vi "Run with Subpanel Settings.vi"(8 "error in (no error)":errorcluster, 11 "VI Refnum In":refnum<vi>) -> (0 "error out":errorcluster, 3 "VI Refnum":refnum<vi>)   [LabVIEW 2021]
doc: "Prepares a VI for running in a subpanel by setting the front panel to origin and hiding the scrollbars, then runs the VI."
uses:
  <vilib>/Utility/miscctls.llb/LVPointTypeDef.ctl
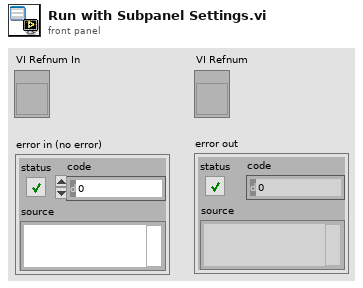
[diagram p1: front panel]
types:
  T1 = typedef "LVPointTypeDef.ctl" = cluster{"Horizontal":i16, "Vertical":i16}
  T2 = enum16{"Always On", "Always Off", "Off While Running"}
  T3 = enum32{"Invalid", "Standard", "Closed", "Hidden", "Minimized", "Maximized"}
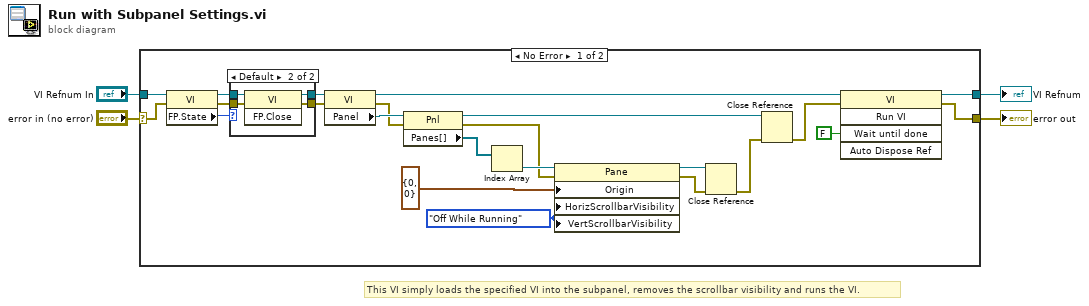
[diagram p0: block diagram]
diagram:
  # "This VI simply loads the specified VI into the subpanel, removes the scrollbar visibility and runs the VI."
  n1 = case shown="No Error" "error in (no error)" {
    selector: "error in (no error)" -> [w8 w34]
    tunnel: "VI Refnum In" -> [w9 w35]
    tunnel: [w13 w35] -> w2
    tunnel: [w12 w34] -> w1
    frame No Error {
      w22 = T2."Off While Running" ("Vertical Scrollbar Visibility")
      n2 = property class="VI"(reference=w9, error in=w8) -> (reference out=w6:refnum<vi>, error out=w5:errorcluster, "FP.State"=w7:T3)
      n3 = case shown="Default" w7 {
        tunnel: [w29 w33] -> w11
        tunnel: [w28 w32] -> w10
        tunnel: w6 -> [w29 w31]
        tunnel: w5 -> [w28 w30]
        frame "Closed" {
        }
        frame Default {
          n4 = invoke class="VI" method="FP.Close"(reference=w31, error in=w30) -> (reference out=w33:refnum<vi>, error out=w32:errorcluster)  [unwired: 1 in, 1 out]
        }
      }
      n5 = property class="VI"(reference=w11, error in=w10) -> (reference out=w16:refnum<vi>, error out=w26:errorcluster, "Panel"=w27:refnum<vi>)
      n6 = property class="Pnl"(reference=w27, error in=w26) -> (reference out=w20:refnum<vi>, error out=w23:errorcluster, "Panes[]"=w25:refnum<vi>[])
      n7 = Index Array(array=w25) -> (element=w24:refnum<vi>)  [unwired: 1 in]
      n8 = property class="Pane"(reference=w24, error in=w23, "Origin"=T1 {"Horizontal"=0, "Vertical"=0}, "HorizScrollbarVisibility"=w22, "VertScrollbarVisibility"=w22) -> (reference out=w19:refnum<vi>, error out=w18:errorcluster)
      n9 = Close Reference(reference=w19, error in (no error)=w18) -> (error out=w17:errorcluster)
      n10 = Close Reference(reference=w20, error in (no error)=w17) -> (error out=w15:errorcluster)
      n11 = invoke class="VI" method="Run VI"(reference=w16, error in=w15, "Wait until done"=FALSE ("Wait Until Done")) -> (reference out=w13:refnum<vi>, error out=w12:errorcluster)  [unwired: 2 in, 3 out]
    }
    frame Error {
    }
  }
  "VI Refnum" <- w2
  "error out" <- w1
